vi "Actor Core.vi"(8 "error in":errorcluster, 11 "Small Panel Actor in":refnum<class "Small Panel Actor.lvclass">) -> (0 "error out":errorcluster, 3 "Actor out":refnum<class "Actor.lvclass">)   [LabVIEW 2013, in "Small Panel Actor.lvlib" / "Small Panel Actor.lvclass"]
doc: "(<B>Filename</B>: Actor Framework.lvlib:Actor.lvclass:Actor Core.vi)\n\nReceives messages to the actor, reacts to them, and initiates any error handling that may shut the actor down.\n\nDescendant classes may override this VI to append parallel tasks for the actor to complete while it handles messages. Overrides use the Call Parent Method node."
uses:
  Small Panel Actor.lvclass
  <vilib>/ActorFramework/Actor/Actor.lvclass
  Reusable/Xctls/Configurable Buffer/Configurable Buffer.xctl
panel:
  in  "Configurable Buffer":cluster{"Val":dbl[], "time":timestamp}(xcontrol)
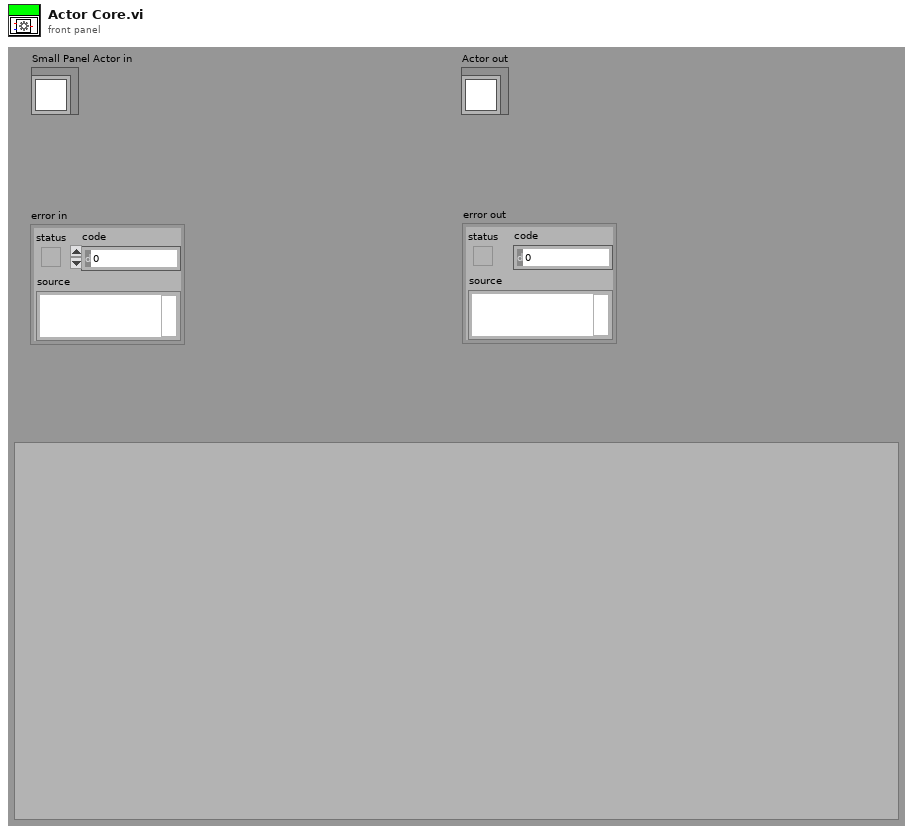
[diagram p1: front panel]
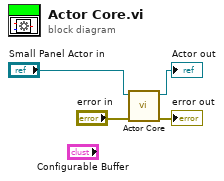
[diagram p0: block diagram]
diagram:
  n1 = call-parent "Actor Core.vi"("error in"="error in", "Actor in"="Small Panel Actor in") -> ("error out"=→"error out":errorcluster, "Actor out"=→"Actor out":refnum<class "Actor.lvclass">)  [unwired: 8 in]
